vi "Sets_Intersect(TimeStamp).vi"(8 "error in (no error)":errorcluster caption="错误输入（无错误）", 10 "输入数组B":timestamp[](array[timestamp]), 11 "输入数组A":timestamp[](array[timestamp])) -> (0 "error out":errorcluster caption="错误输出", 3 "输出数组C":timestamp[](array[timestamp]))   [LabVIEW 2012]
uses:
  Sets_Unique(TimeStamp).vi
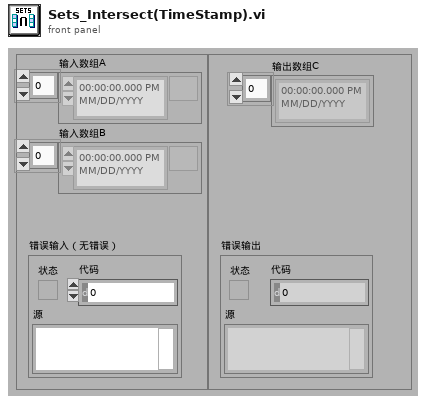
[diagram p1: front panel]
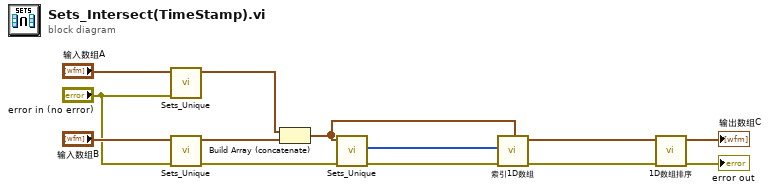
[diagram p0: block diagram]
diagram:
  n1 = call-poly "Sets_Unique.vi"("error in (no error)"="error in (no error)", "输入数组"="输入数组A") -> ("输出数组"=w4:timestamp[])  [unwired: 7 in, 2 out]
  n2 = call-poly "Sets_Unique.vi"("error in (no error)"="error in (no error)", "输入数组"="输入数组B") -> ("error out"=w12:errorcluster, "输出数组"=w3:timestamp[])  [unwired: 7 in, 1 out]
  n3 = Build Array (concatenate)(w4, w3) -> (w6:timestamp[])
  n4 = call-poly "Sets_Unique.vi"("error in (no error)"=w12, "输入数组"=w6) -> ("error out"=w9:errorcluster, "已删除元素索引"=w7:i32[])  [unwired: 7 in, 1 out]
  n5 = call-poly "索引1D数组.vi"("error in (no error)"=w9, "索引"=w7, "输入数组"=w6) -> ("error out"=w8:errorcluster, "元素"=w2:timestamp[])  [unwired: 7 in]
  n6 = call-poly "1D数组排序.vi"("error in (no error)"=w8, "输入数组"=w2) -> ("error out"=→"error out":errorcluster, "排序后数组"=→"输出数组C":timestamp[])  [unwired: 7 in, 1 out]
